vi "CSDB_Common.MySelect.vi"(5 "optional clause":string, 6 "error in (no error)":errorcluster, 7 "column":string, 8 "table":string, 9 "connection reference":T1) -> (0 "error out":errorcluster, 1 "1d output array":string[](array[string]), 3 "connection reference out":T1)   [LabVIEW 2014, in "CSDB_Common.lvlib"]
doc: "This Vi uses the \"DB Tools Select Data\" to pick data from one single column in a 1-D array."
uses:
  CSDB_Common.lvlib
  <vilib>/addons/database/Connection.llb/Conn ObjectReference.ctl
  <vilib>/addons/database/NI_Database_API.lvlib
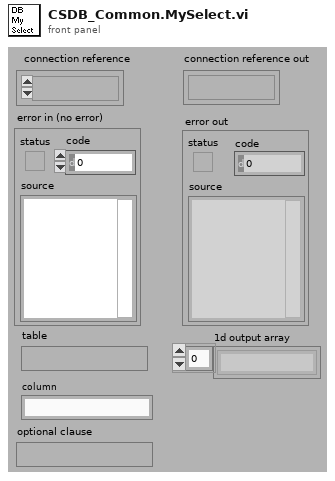
[diagram p1: front panel]
types:
  T1 = typedef "NI_Database_API.lvlib/Conn ObjectReference.ctl" = refnum<k1>
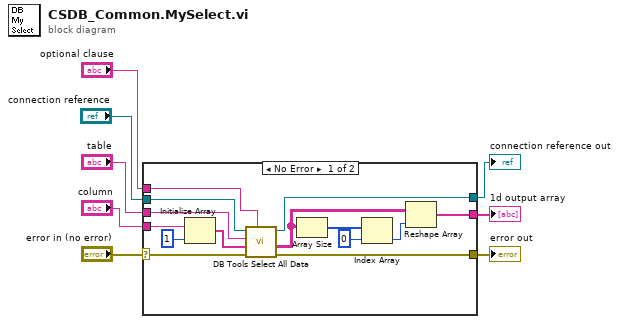
[diagram p0: block diagram]
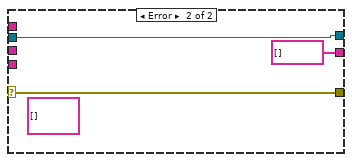
[diagram p2: hidden frame]
diagram:
  n1 = case shown="No Error" "error in (no error)" {
    selector: "error in (no error)" -> [w11 w25]
    tunnel: "column" -> [w22 _]
    tunnel: [w19 string[] [] ("data")] -> w7
    tunnel: "connection reference" -> [w18 w24]
    tunnel: "table" -> [w17 _]
    tunnel: [w15 w24] -> w4
    tunnel: [w14 w25] -> w3
    tunnel: "optional clause" -> [w9 _]
    frame No Error {
      n2 = Initialize Array(w22, 1 ("dimension size")) -> (w16:string[])
      n3 = call <vilib>:"DB Tools Select All Data.vi"("optional clause"=w9, "error in (no error)"=w11, "columns"=w16, "table"=w17, "connection reference"=w18) -> ("error out"=w14:errorcluster, "data"=w10:string[][], "connection reference out"=w15:T1)  [unwired: 1 in]
      n4 = Array Size(array=w10) -> (size(s)=w13:i32[])
      n5 = Index Array(array=w13, index=0) -> (element=w12:i32)
      n6 = Reshape Array(w10, w12) -> (w19:string[])
    }
    frame Error {
      (unwired) string[][] [] ("data")
    }
  }
  "connection reference out" <- w4
  "error out" <- w3
  "1d output array" <- w7
